vi "搜索所有匹配元素(1D CDB).vi"(8 "error in (no error)":errorcluster caption="错误输入（无错误）", 9 "开始索引（0）":i32, 10 "元素":cdb, 11 "数组":cdb[](array[numeric])) -> (0 "error out":errorcluster caption="错误输出", 1 "匹配数量":i32, 3 "匹配元素索引":i32[](array[numeric]))   [LabVIEW 2012]
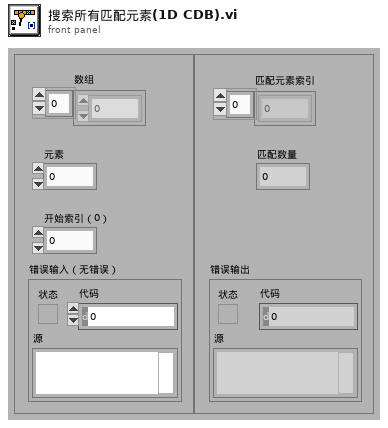
[diagram p1: front panel]
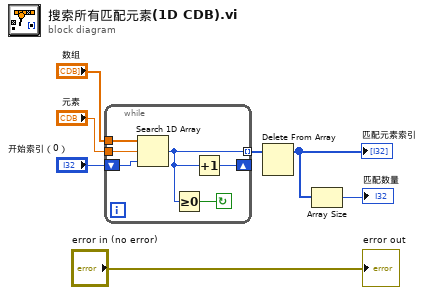
[diagram p0: block diagram]
diagram:
  n1 = while {
    tunnel: "数组" -> [w13]
    tunnel: "元素" -> [w12]
    shift-right: [w9] -> _
    shift-left: "开始索引（0）" -> [w11]
    tunnel: [w8] -> w4 mode=indexing
    stop <- w10 continue-if-true
    n2 = Search 1D Array(1D array=w13, element=w12, start index (0)=w11) -> (index of element=w8:i32)
    n3 = Greater Or Equal To 0?(x=w8) -> (x >= 0?=w10:bool)
    n4 = Increment(x=w8) -> (x+1=w9:i32)
  }
  n5 = Delete From Array(array=w4) -> (array with subset deleted=w2:i32[])  [unwired: 2 in, 1 out]
  "匹配元素索引" <- w2
  n6 = Array Size(array=w2) -> (size(s)=→"匹配数量":i32)
  "error out" <- "error in (no error)"
